vi "ExSubReadFrameFromFile.vi"(2 "error in (no error)":errorcluster, 3 "Frame to pull off":u32, 4 "File type":u32, 5 "path to file to open":path) -> (0 "error out":errorcluster, 1 "Image Handle":u32)   [LabVIEW 2010]
panel:
  # "ExSubReadFrameFromFile.vi:\nThis sub VI takes a file type\nand path with file name and a \nframe number to pull off and \nthen returns an image handle\nwith that frame read from file."
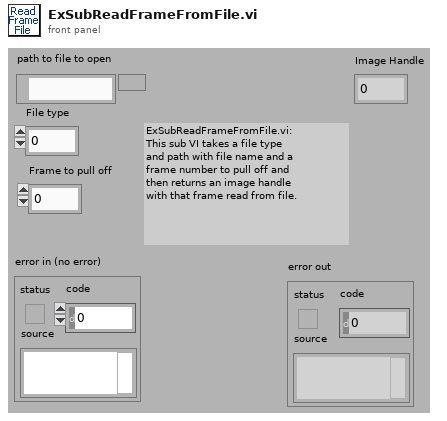
[diagram p1: front panel]
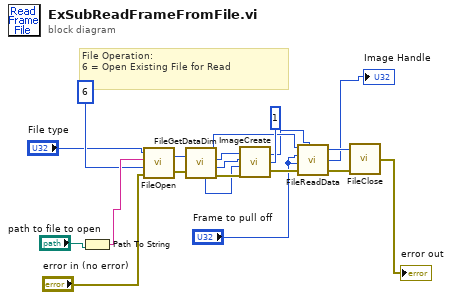
[diagram p0: block diagram]
diagram:
  # "File Operation:\n6 = Open Existing File for Read"
  n1 = Path To String(path="path to file to open") -> (string=w7:string)
  n2 = call <userlib>:"FileOpen.vi"("error in"="error in (no error)", "File Operations"=u32 6 ("File Operation"), "FileName"=w7, "File Type"="File type") -> ("error out"=w20:errorcluster, "File Handle"=w19:u32)
  n3 = call <userlib>:"FileGetDataDim.vi"("File Handle"=w19, "error in"=w20) -> ("Data Type"=w17:u32, "File Handle"=w13:u32, "X dim"=w10:u32, "Y dim"=w11:u32, "error out"=w18:errorcluster)  [unwired: 1 out]
  n4 = call <userlib>:"ImageCreate.vi"("X dimension"=w10, "Y dimension"=w11, "Data Type"=w17, "error in"=w18, "Number Of Frames"=1) -> ("Image Handle"=w9:u32, "error out"=w15:errorcluster)
  n5 = call <userlib>:"FileReadData.vi"("File Handle"=w13, "Start Frame"="Frame to pull off", "End Frame"="Frame to pull off", "error in"=w15, "Image Handle"=w9) -> ("File Handle"=w12:u32, "Image Handle"=→"Image Handle":u32, "error out"=w14:errorcluster)
  n6 = call <userlib>:"FileClose.vi"("error in"=w14, "File Handle"=w12) -> ("error out"=→"error out":errorcluster)
